vi "Server_Main Initialize.vi"(8 "error in":errorcluster, 11 "VI Reference":refnum<vi>) -> (0 "error out":errorcluster)   [LabVIEW 2018, in "Cloud Server.lvlib"]
doc: "進行伺服器主程式的初始化。"
uses:
  Cloud Server.lvlib
  Data Def/Server_Error Handle Method.ctl
  Data Def/Server_FGV Method.ctl
  Data Def/Server_Connection Manager Method.ctl
  Com VIs/Data Def/stm_MetaElement.ctl
  Com VIs/Data Def/stm_MetaDataElement.ctl
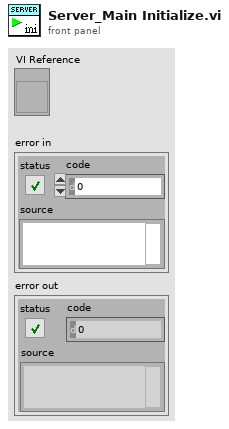
[diagram p1: front panel]
types:
  T1 = typedef "Cloud Server.lvlib/Server_Error Handle Method.ctl" = enum16{"Initialize", "Get Queue Ref.", "Enqueue", "Insert", "Flush", "Release"}
  T2 = typedef "Cloud Server.lvlib/Server_FGV Method.ctl" = enum16{"Get", "Put"}
  T3 = typedef "Cloud Server.lvlib/Server_Connection Manager Method.ctl" = enum16{"Initialize", "Add", "Get", "Set Properties", "Get Properties", "Close", "Release"}
  T4 = typedef "Cloud Server.lvlib/Server_Main Data.ctl" = cluster{"Main VI Ref.":refnum<vi>, "Listener ID":refnum<k5>, "Meta data":T5[], "Main Queue":T7, "User Picture":T8}
  T5 = typedef "stm_MetaElement.ctl" = cluster{"Name":T6}
  T6 = typedef "stm_MetaDataElement.ctl" = string
  T7 = typedef "Cloud Server.lvlib/Server_Main Queue.ctl" = cluster{"Server Write Queue":refnum<queue>, "Main Loop Queue":refnum<queue>}
  T8 = typedef "IMAQ Image.ctl" = refnum<image>
  T9 = typedef "Image Type" = u32
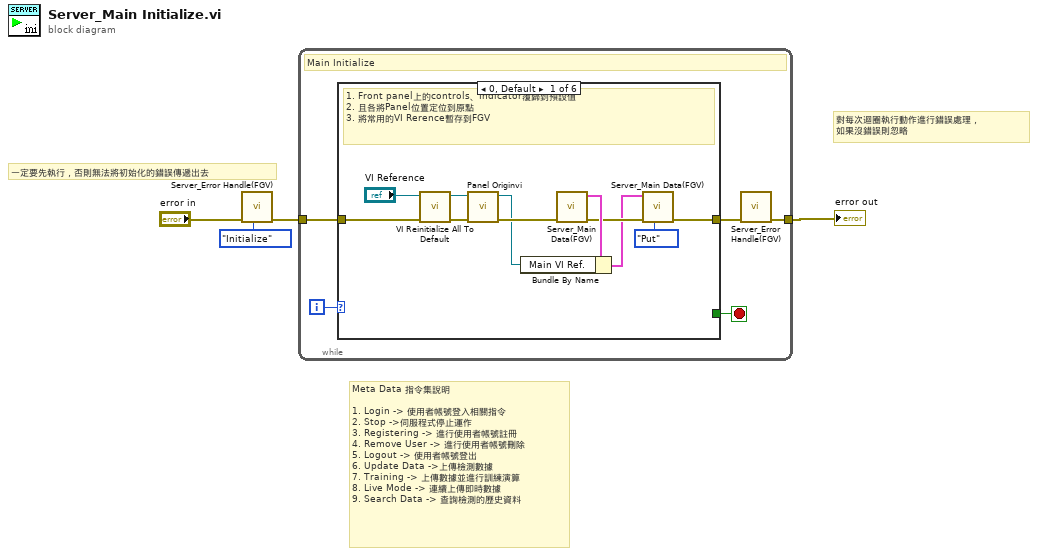
[diagram p0: block diagram]
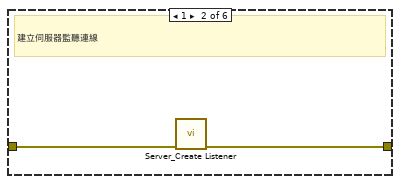
[diagram p2: hidden frame]
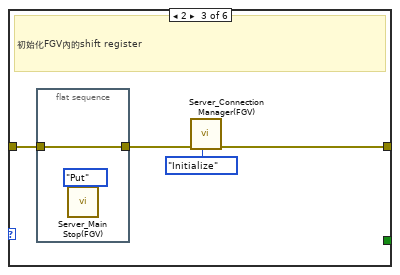
[diagram p3: hidden frame]
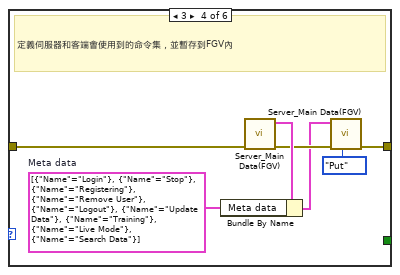
[diagram p4: hidden frame]
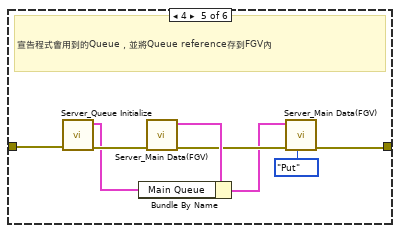
[diagram p5: hidden frame]
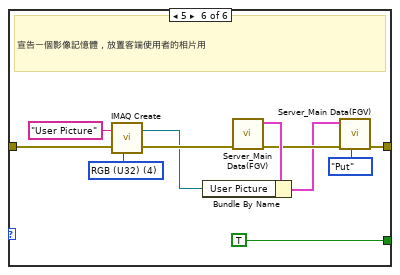
[diagram p6: hidden frame]
diagram:
  # "Meta Data 指令集說明\n\n1. Login -> 使用者帳號登入相關指令\n2. Stop ->伺服程式停止運作\n3. Registering -> 進行使用者帳號註冊\n4. Remove User -> 進行使用者帳號刪除\n5. Logout -> 使用者帳號登出\n6. Update Data ->上傳檢測數據\n7. Training -> 上傳數據並進行訓練演算\n8. Live Mode -> 連續上傳即時數據\n9. Search Data -> 查詢檢測的歷史資料"
  # "對每次迴圈執行動作進行錯誤處理，\n如果沒錯誤則忽略"
  # "一定要先執行，否則無法將初始化的錯誤傳遞出去"
  n1 = call "Server_Error Handle(FGV).vi"("Error Handle Method(Enqueue)"=Server_Error_Handle_Method."Initialize" ("Error Handle Method"), "error in"="error in") -> ("error out"=w3:errorcluster)  [unwired: 8 in, 1 out]
  n2 = while {
    tunnel: w3 -> [w8]
    tunnel: [w6] -> w1
    i -> [w9]
    stop <- w5 stop-if-true
    # "Main Initialize"
    n3 = case shown="0, Default" w9 {
      tunnel: w8 -> [w17 w22 w26 w31 w43 w51]
      tunnel: [w12 w21 w24 w30 w36 w45] -> w7
      tunnel: [_ _ _ _ _ TRUE] -> w5
      frame 0, Default {
        # "1. Front panel上的controls、Indicator覆歸到預設值\n2. 且各將Panel位置定位到原點\n3. 將常用的VI Rerence暫存到FGV"
        n4 = call "VI Reinitialize All To Default.vi"("error in"=w17, "VI Reference in"="VI Reference") -> ("error out"=w20:errorcluster, "VI Reference out"=w19:refnum<vi>)  [unwired: 8 in]
        n5 = call "Panel Originvi.vi"("error in"=w20, "VI Reference In"=w19) -> ("error out"=w16:errorcluster, "VI Reference Out"=w14:refnum<vi>)  [unwired: 8 in]
        n6 = call "Server_Main Data(FGV).vi"("error in"=w16) -> ("error out"=w13:errorcluster, "Main Data Out"=w15:T4)  [unwired: 9 in]
        n7 = Bundle By Name(cluster=w15, "Main VI Ref."=w14) -> (w11:T4)
        n8 = call "Server_Main Data(FGV).vi"("FGV Method(Get)"=Server_FGV_Method."Put", "error in"=w13, "Main Data In"=w11) -> ("error out"=w12:errorcluster)  [unwired: 7 in, 1 out]
      }
      frame 1 {
        # "建立伺服器監聽連線"
        n9 = call "Server_Create Listener.vi"("error in"=w22) -> ("error out"=w21:errorcluster)  [unwired: 10 in]
      }
      frame 2 {
        # "初始化FGV內的shift register"
        n10 = flat-sequence {
          tunnel: w26 -> [w27]
          tunnel: [w27] -> w25
          frame #0 {
            n11 = call "Server_Main Stop(FGV).vi"("FGV Method"=Server_FGV_Method."Put") -> ()  [unwired: 3 in, 1 out]
          }
        }
        n12 = call "Server_Connection Manager(FGV).vi"("Connection Manager Method(Get)"=Server_Connection_Manager_Method."Initialize", "error in"=w25) -> ("error out"=w24:errorcluster)  [unwired: 5 in, 4 out]
      }
      frame 3 {
        w29 = T5[] [{"Name"="Login"}, {"Name"="Stop"}, {"Name"="Registering"}, {"Name"="Remove User"}, {"Name"="Logout"}, {"Name"="Update Data"}, {"Name"="Training"}, {"Name"="Live Mode"}, {"Name"="Search Data"}]  # Meta data
        # "定義伺服器和客端會使用到的命令集，並暫存到FGV內"
        n13 = call "Server_Main Data(FGV).vi"("error in"=w31) -> ("error out"=w34:errorcluster, "Main Data Out"=w35:T4)  [unwired: 9 in]
        n14 = Bundle By Name(cluster=w35, "Meta data"=w29) -> (w33:T4)
        n15 = call "Server_Main Data(FGV).vi"("FGV Method(Get)"=Server_FGV_Method."Put", "error in"=w34, "Main Data In"=w33) -> ("error out"=w30:errorcluster)  [unwired: 7 in, 1 out]
      }
      frame 4 {
        # "宣告程式會用到的Queue，並將Queue reference存到FGV內"
        n16 = call "Server_Queue Initialize.vi"("error in"=w43) -> ("error out"=w42:errorcluster, "Main Queue"=w40:T7)  [unwired: 9 in]
        n17 = call "Server_Main Data(FGV).vi"("error in"=w42) -> ("error out"=w39:errorcluster, "Main Data Out"=w41:T4)  [unwired: 9 in]
        n18 = Bundle By Name(cluster=w41, "Main Queue"=w40) -> (w38:T4)
        n19 = call "Server_Main Data(FGV).vi"("FGV Method(Get)"=Server_FGV_Method."Put", "error in"=w39, "Main Data In"=w38) -> ("error out"=w36:errorcluster)  [unwired: 7 in, 1 out]
      }
      frame 5 {
        w52 = T9 4 items=["Grayscale (U8)", "Grayscale (I16)", "Grayscale (SGL)", "Complex (CSG)", "RGB (U32)", "HSL (U32)", "RGB (U64)", "Grayscale (U16)"] ("Image Type")
        # "宣告一個影像記憶體，放置客端使用者的相片用"
        n20 = call "IMAQ Create"("Image Name"="User Picture", "Image Type"=w52, "error in (no error)"=w51) -> ("New Image"=w44:T8, "error out"=w46:errorcluster)  [unwired: 2 in]
        n21 = call "Server_Main Data(FGV).vi"("error in"=w46) -> ("error out"=w49:errorcluster, "Main Data Out"=w50:T4)  [unwired: 9 in]
        n22 = Bundle By Name(cluster=w50, "User Picture"=w44) -> (w48:T4)
        n23 = call "Server_Main Data(FGV).vi"("FGV Method(Get)"=Server_FGV_Method."Put", "error in"=w49, "Main Data In"=w48) -> ("error out"=w45:errorcluster)  [unwired: 7 in, 1 out]
      }
    }
    n24 = call "Server_Error Handle(FGV).vi"("error in"=w7) -> ("error out"=w6:errorcluster)  [unwired: 9 in, 1 out]
  }
  "error out" <- w1
